vi "EXAMPLE_REF.vi"() -> ()   [LabVIEW 2017]
uses:
  ed4e8434-f5d1-4aa9-a705-4eb138cf39a7.vi
  1c0b7591-5e20-4383-a033-ad08ad6277ea.vi
  966f5005-d432-4239-b76d-566671f38609.vi
  e168b5b1-2942-41e2-994e-ab5d1da95eb0.vi
  2714d762-8b69-473d-9a97-9be709e3a6d3.vi
  fbb81e0b-51e1-459c-8863-f1499de531db.vi
  225ae018-2966-4a81-bc75-f762216825e6.vi
  TagDB/_Support/Error/_Clear Errors.vi
  TagDB/_Support/DataType/_dataType.vi
  TagDB/_Support/DataType/_refNumType.vi
  ed4e8434-f5d1-4aa9-a705-4eb138cf39a7.vi/8f6460cc-fc72-4ccc-8f3c-e93b8a5372ad.vi
  1c0b7591-5e20-4383-a033-ad08ad6277ea.vi/69f1a093-ef09-4560-8ba1-dc8c689b3bf0.vi
  966f5005-d432-4239-b76d-566671f38609.vi/8f6460cc-fc72-4ccc-8f3c-e93b8a5372ad.vi
  e168b5b1-2942-41e2-994e-ab5d1da95eb0.vi/69f1a093-ef09-4560-8ba1-dc8c689b3bf0.vi
  2714d762-8b69-473d-9a97-9be709e3a6d3.vi/8f6460cc-fc72-4ccc-8f3c-e93b8a5372ad.vi
  fbb81e0b-51e1-459c-8863-f1499de531db.vi/90410410-40ef-4a1e-92ae-bfc967ad4294.vi
  TagDB/API/TagDB-Status.vi
  225ae018-2966-4a81-bc75-f762216825e6.vi/90410410-40ef-4a1e-92ae-bfc967ad4294.vi
  TagDB/_Support/DataAccess/_NameCacher.vi
  TagDB/_Support/DataAccess/_datatypeChecker.vi
  TagDB/_Support/DataAccess/TagDB Ref to DVR.vi
  <vilib>/Utility/Data Type/Get Type Information.vi
  <vilib>/Utility/error.llb/Trim Whitespace.vi
  TagDB/_Support/Error/_[error50000]Invalid DB REF.vi
  TagDB/_Support/Change Detector/TagDB dbChanged.vi
  TagDB/_Support/Error/_[error50002]Invalid DataType.vi
  TagDB/TagDB.lvlib
panel:
  out "Array 2":dbl[](array[numeric])=[123.0]
  out "Array":string[](array[string])=["Numeric0", "Numeric1"]
  in  "Numeric1":string="abc"
  out "Value 0":dbl=123.0
  out "Class Name":string="Digital"
  in  "Numeric0":dbl=123.0
  out "label":string="Numeric0"
  # "1"
  # "2"
  # "3"
  # "4"
  # "5"
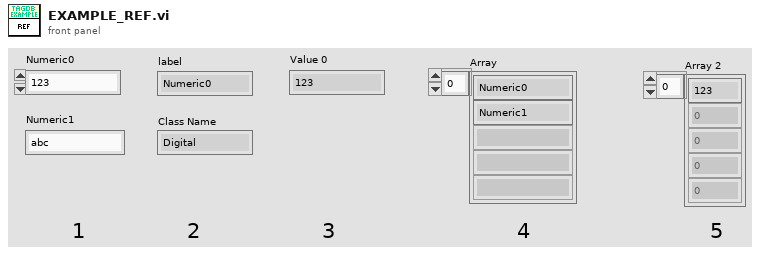
[diagram p1: front panel]
types:
  T1 = typedef "TagDB.lvlib/TagDB.ctl" = refnum<k1>
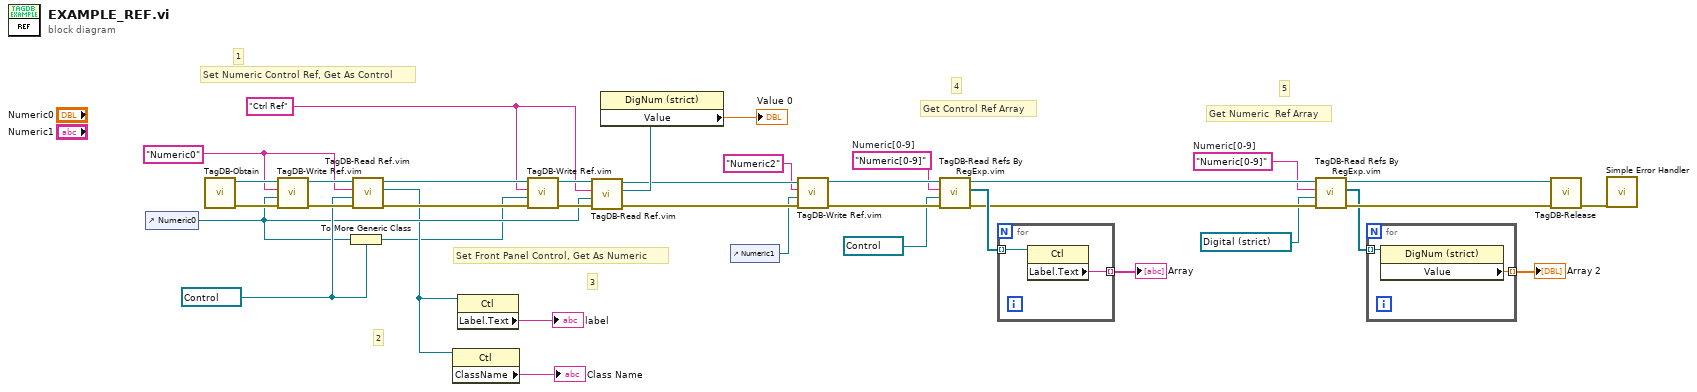
[diagram p0: block diagram]
diagram:
  w2 = "Numeric[0-9]"  # Numeric[0-9]
  w3 = "Numeric[0-9]"  # Numeric[0-9]
  w27 = "Ctrl Ref"
  w25 = refnum<vi> refnum ("value")
  w34 = "Numeric0"
  # "5"
  # "4"
  # "1"
  # "3"
  # "2"
  # "Get Numeric  Ref Array"
  # "Get Control Ref Array"
  # "Set Front Panel Control, Get As Numeric"
  # "Set Numeric Control Ref, Get As Control"
  n1 = control-ref of="Numeric0"() -> (w23:refnum<vi>)
  n2 = call "TagDB-Obtain.vi"() -> ("error out"=w35:errorcluster, "TagDB"=w36:T1)  [unwired: 5 in, 1 out]
  n3 = call "TagDB-Write Ref.vim"("Error In"=w35, "value"=w23, "name"=w34, "DB Ref"=w36) -> ("Error Out"=w33:errorcluster, "DB Ref(dup)"=w37:T1)  [unwired: 5 in, 1 out]
  n4 = To More Generic Class(target class=w25, reference=w23) -> (generic class reference=w1:refnum<vi>)
  n5 = call "TagDB-Read Ref.vim"("error in (no error)"=w33, "Type"=w25, "name"=w34, "DB Ref"=w37) -> ("error out"=w28:errorcluster, "value"=w21:refnum<vi>, "DB Ref(dup)"=w29:T1)  [unwired: 5 in]
  n6 = property class="Ctl"(reference=w21) -> ("ClassName"=→"Class Name":string)  [unwired: 1 in, 2 out]
  n7 = property class="Ctl"(reference=w21) -> ("Label.Text"=→"label":string)  [unwired: 1 in, 2 out]
  n8 = call "TagDB-Write Ref.vim"("Error In"=w28, "value"=w1, "name"=w27, "DB Ref"=w29) -> ("Error Out"=w31:errorcluster, "DB Ref(dup)"=w30:T1)  [unwired: 5 in, 1 out]
  n9 = call "TagDB-Read Ref.vim"("error in (no error)"=w31, "Type"=w23, "name"=w27, "DB Ref"=w30) -> ("error out"=w19:errorcluster, "value"=w24:refnum<vi>, "DB Ref(dup)"=w20:T1)  [unwired: 5 in]
  n10 = property class="DigNum (strict)"(reference=w24) -> ("Value"=→"Value 0":dbl)  [unwired: 1 in, 2 out]
  n11 = control-ref of="Numeric1"() -> (w18:refnum<vi>)
  n12 = call "TagDB-Write Ref.vim"("Error In"=w19, "value"=w18, "name"="Numeric2", "DB Ref"=w20) -> ("Error Out"=w15:errorcluster, "DB Ref(dup)"=w16:T1)  [unwired: 5 in, 1 out]
  n13 = call "TagDB-Read Refs By RegExp.vim"("error in (no error)"=w15, "Type"=refnum<vi> refnum ("value"), "RegExp"=w3, "DB Ref"=w16) -> ("error out"=w8:errorcluster, "value"=w13:refnum<vi>[], "DB Ref(dup)"=w9:T1)  [unwired: 4 in, 1 out]
  n14 = for {
    tunnel: w13 -> [w39] mode=indexing
    tunnel: [w38] -> w12 mode=indexing
    n15 = property class="Ctl"(reference=w39) -> ("Label.Text"=w38:string)  [unwired: 1 in, 2 out]
  }
  "Array" <- w12
  n16 = call "TagDB-Read Refs By RegExp.vim"("error in (no error)"=w8, "Type"=refnum<vi> refnum ("Numeric1"), "RegExp"=w2, "DB Ref"=w9) -> ("error out"=w11:errorcluster, "value"=w7:refnum<vi>[], "DB Ref(dup)"=w10:T1)  [unwired: 4 in, 1 out]
  n17 = for {
    tunnel: w7 -> [w41] mode=indexing
    tunnel: [w40] -> w6 mode=indexing
    n18 = property class="DigNum (strict)"(reference=w41) -> ("Value"=w40:dbl)  [unwired: 1 in, 2 out]
  }
  "Array 2" <- w6
  n19 = call "TagDB-Release.vi"("error in (no error)"=w11, "TagDB"=w10) -> ("error out"=w4:errorcluster)  [unwired: 9 in]
  n20 = call <vilib>:"Simple Error Handler.vi"("error in (no error)"=w4) -> ()  [unwired: 4 in, 5 out]
